vi "processAllFramesMatlab.vi"(1 "cropLinesOut":dbl, 3 "Output Path":path, 4 "Scan":refnum<class "Scan.lvclass">, 6 "Progress":refnum<vi>, 9 "Display":refnum<vi>, 12 "Updated camera":T2, 14 "OCT filename out":string) -> ()   [LabVIEW 2017]
uses:
  <vilib>/vision/Image Controls.llb/IMAQ Image.ctl
  classes/Scans/Scan.lvclass
  classes/HardwareObjects/Camera/Camera.lvclass
  classes/Scans/Scan.lvclass/Scan.ctl
  <vilib>/Analysis/1siggen.llb/Ramp Pattern by Samples.vi
  classes/Scans/Read A scans.vi
  classes/Scans/Read Repeat B scans.vi
  classes/Scans/Read C scans.vi
  classes/Scans/Read B scans.vi
  classes/Scans/Read Total B-Scans.vi
  <vilib>/Analysis/NI_AALBase.lvlib
panel:
  out "Array":dbl[](array[numeric])
  out "Path":path
  in  "Camera in":refnum<class "Camera.lvclass">
  out "oct-a volume out":dbl[][][](array[numeric])
  out "oct volume out":dbl[][][](array[numeric])
  out "xRpt":dbl
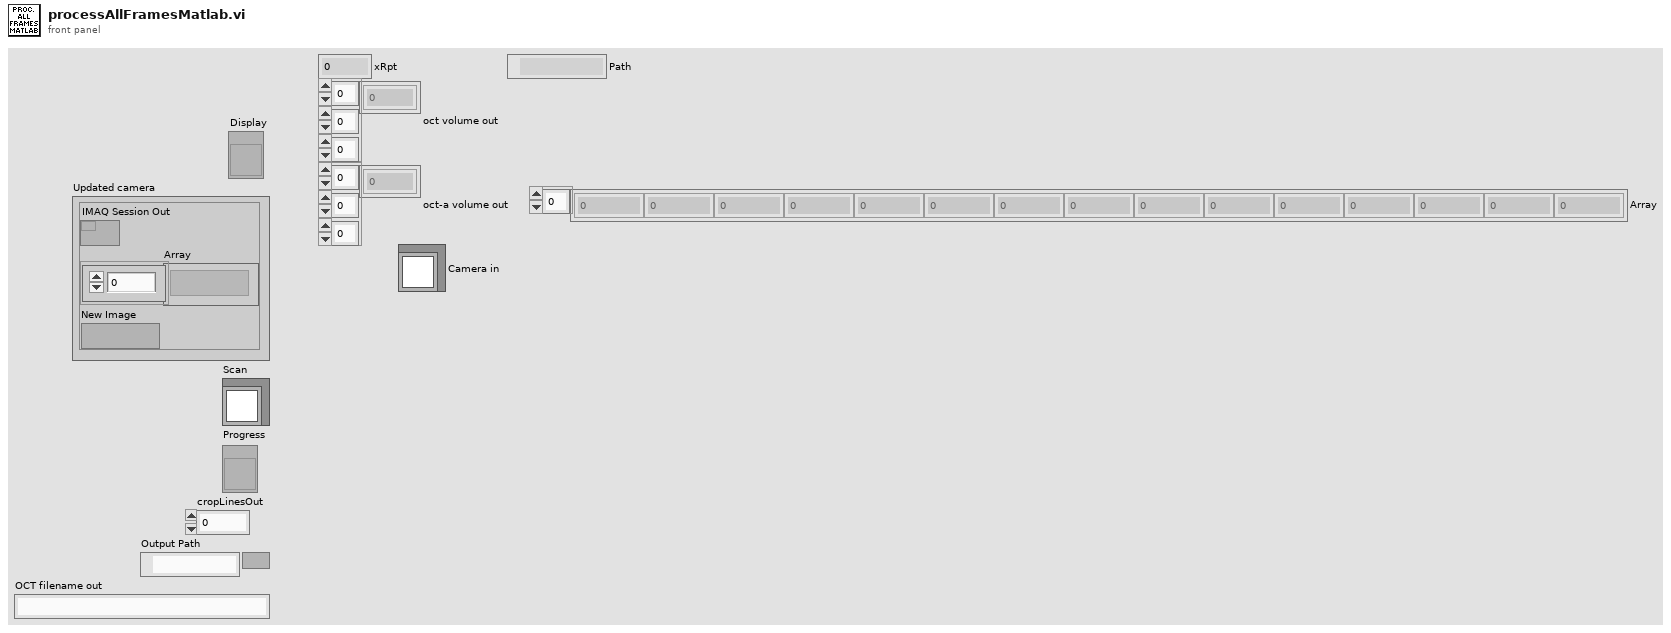
[diagram p1: front panel]
types:
  T1 = typedef "IMAQ Image.ctl" = refnum<image>
  T2 = cluster{"IMAQ Session Out":refnum<k11>, "Array":T1[], "New Image":T1}
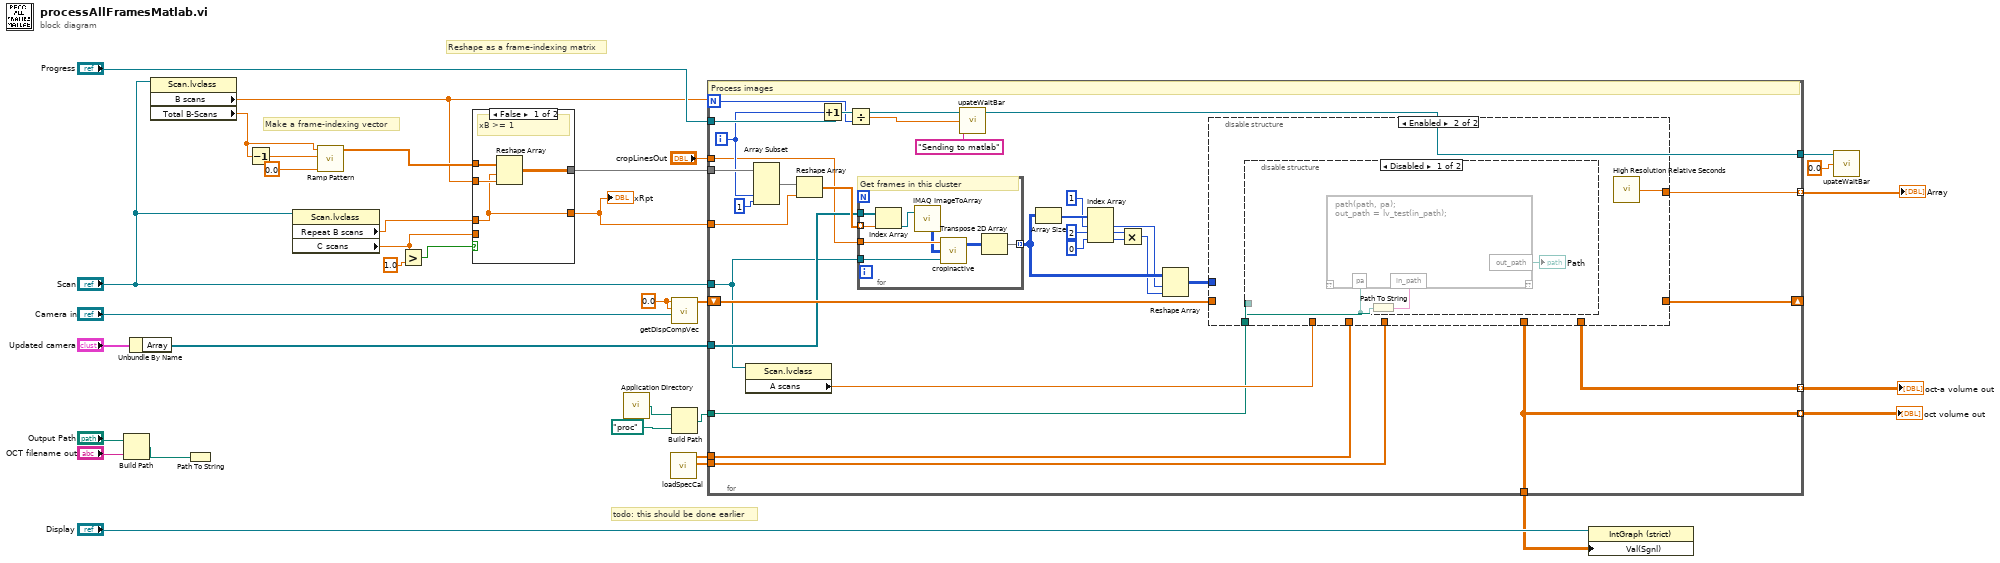
[diagram p0: block diagram]
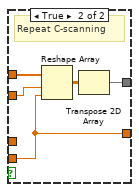
[diagram p2: hidden frame]
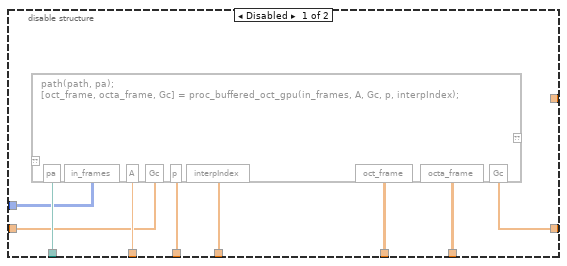
[diagram p3: hidden frame]
diagram:
  w4 = 0.0 ("C2")
  # "Reshape as a frame-indexing matrix"
  # "todo: this should be done earlier"
  # "Make a frame-indexing vector"
  n1 = Build Path(base path="Output Path", name or relative path="OCT filename out") -> (appended path=w25:path)
  n2 = Unbundle By Name("Updated camera") -> ("Array"=w32:T1[])
  n3 = property class="Scan.lvclass"(reference="Scan") -> ("B scans"=w9:dbl, "Total B-Scans"=w17:dbl)  [unwired: 1 in, 2 out]
  n4 = Path To String(path=w25) -> ()  [unwired: 1 out]
  n5 = Decrement(x=w17) -> (x-1=w18:dbl)
  n6 = property class="Scan.lvclass"(reference="Scan") -> ("Repeat B scans"=w10:dbl, "C scans"=w11:dbl)  [unwired: 1 in, 2 out]
  n7 = call-poly <vilib>:"Ramp Pattern.vi"("start"=0.0, "end"=w18, "samples"=w17) -> ("Ramp Pattern"=w14:dbl[])  [unwired: 7 in, 1 out]
  n8 = Greater?(x=w11, y=1.0) -> (0:w12:bool)
  n9 = case shown="False" w12 {
    tunnel: w14 -> [w38 w43]
    tunnel: [w36 w40] -> w13
    tunnel: w11 -> [_ w39]
    tunnel: w10 -> [w35 _]
    tunnel: w9 -> [w37 w42]
    tunnel: [w35 w39] -> w8
    frame False {
      # "xB >= 1"
      n10 = Reshape Array(w38, w35, w37) -> (w36:dbl[][])
    }
    frame True {
      # "Repeat C-scanning"
      n11 = Reshape Array(w43, w42, w39) -> (w41:dbl[][])
      n12 = Transpose 2D Array(2D array=w41) -> (transposed array=w40:dbl[][])
    }
  }
  "xRpt" <- w8
  n13 = call <vilib>:"Application Directory.vi"() -> ("Application Directory"=w22:path)
  n14 = call "loadSpecCal.vi"() -> ("interp_index"=w23:dbl[], "P"=w24:dbl[])  [unwired: 10 in]
  n15 = call "getDispCompVec.vi"("Camera in"="Camera in", "C3"=w4, "C2"=w4) -> ("Gc"=w2:cdb[])  [unwired: 8 in]
  n16 = Build Path(base path=w22, name or relative path=path "proc") -> (appended path=w20:path)
  n17 = for {
    N: w9 -> [w72]
    tunnel: w32 -> [w59]
    tunnel: "Scan" -> [w57]
    tunnel: "Progress" -> [w77]
    tunnel: [w73] -> w30
    tunnel: "cropLinesOut" -> [w58]
    tunnel: w24 -> [w67]
    tunnel: w23 -> [w66]
    tunnel: w20 -> [w70]
    shift-right: [w69] -> _
    shift-left: w2 -> [w68]
    tunnel: w13 -> [w65]
    tunnel: w8 -> [w61]
    tunnel: [w45] -> w7 mode=indexing
    tunnel: [w46] -> w6 mode=indexing
    tunnel: [w45] -> w5
    tunnel: [w44] -> w1 mode=indexing
    i -> [w64]
    # "Process images"
    n18 = property class="Scan.lvclass"(reference=w57) -> ("A scans"=w71:dbl)  [unwired: 1 in, 2 out]
    n19 = Array Subset(array=w65, index (col)=w64, length (col)=1 ("length")) -> (w62:dbl[][])  [unwired: 2 in]
    n20 = Reshape Array(w62, w61) -> (w60:dbl[])
    n21 = Increment(x=w64) -> (x+1=w76:i32)
    n22 = Divide(x=w76, y=w72) -> (x/y=w75:dbl)
    n23 = for {
      tunnel: w60 -> [w98] mode=indexing
      tunnel: w59 -> [w99]
      tunnel: w58 -> [w96]
      tunnel: w57 -> [w94]
      tunnel: [w92] -> w56 mode=indexing
      # "Get frames in this cluster"
      n24 = Index Array(array=w99, index=w98) -> (element=w97:T1)
      n25 = call "IMAQ ImageToArray"("Image"=w97) -> ("Image Pixels (U16)"=w95:u16[][])  [unwired: 3 in, 4 out]
      n26 = call "cropInactive.vi"("Scan in"=w94, "Whole camera frame"=w95, "cropLines"=w96) -> ("Cropped camera frame"=w93:u16[][])  [unwired: 1 in]
      n27 = Transpose 2D Array(2D array=w93) -> (transposed array=w92:u16[][])
    }
    n28 = call "upateWaitBar.vi"("waitbar text"="Sending to matlab", "waitbar value [0,1]"=w75, "Progress"=w77) -> ("Updated Progress"=w73:refnum<vi>)  [unwired: 2 in]
    n29 = Array Size(array=w56) -> (size(s)=w55:i32[])
    n30 = Index Array(array=w55, index #1=1 ("index"), index #2=2 ("index"), index #3=0 ("index")) -> (element #1=w53:i32, element #2=w50:i32, element #3=w49:i32)
    n31 = Multiply(x=w50, y=w49) -> (x*y=w48:i32)
    n32 = Reshape Array(w56, w53, w48) -> (w47:u16[][])
    n33 = disable-structure shown="Enabled" {
      disable-tunnel: w71 -> [w86 _]
      disable-tunnel: w70 -> [w85 w88]
      disable-tunnel: [w84 _] -> w69
      disable-tunnel: w68 -> [w83 _]
      disable-tunnel: w67 -> [w82 _]
      disable-tunnel: w66 -> [w81 _]
      disable-tunnel: w47 -> [w80 _]
      disable-tunnel: [w79 _] -> w46
      disable-tunnel: [w78 _] -> w45
      disable-tunnel: [_ w87] -> w44
      frame Disabled {
        n34 = script code="path(path, pa);\n[oct_frame, octa_frame, Gc] = proc_buffered_oct_gpu(in_frames, A, Gc, p, interpIndex);"("pa"=w85, "in_frames"=w80, "Gc"=w83, "A"=w86, "p"=w82, "interpIndex"=w81) -> ("oct_frame"=w78:dbl[][], "Gc"=w84:cdb[], "octa_frame"=w79:dbl[][])  [unwired: 1 in, 1 out]
      }
      frame Enabled {
        n35 = disable-structure shown="Disabled" {
          disable-tunnel: w88 -> [w90 _]
          frame Disabled {
            n36 = Path To String(path=w90) -> (string=w91:string)
            n37 = script code="path(path, pa);\nout_path = lv_test(in_path);"("in_path"=w91, "pa"=w90) -> ("out_path"=→"Path":path)  [unwired: 1 in, 1 out]
          }
          frame Enabled {
          }
        }
        n38 = call <vilib>:"High Resolution Relative Seconds.vi"() -> ("relative seconds"=w87:dbl)
      }
    }
  }
  "oct volume out" <- w7
  "oct-a volume out" <- w6
  "Array" <- w1
  n39 = property class="IntGraph (strict)"(reference="Display", "Val(Sgnl)"=w5) -> ()  [unwired: 1 in, 2 out]
  n40 = call "upateWaitBar.vi"("waitbar value [0,1]"=sgl 0.0, "Progress"=w30) -> ()  [unwired: 3 in, 1 out]
